vi "IntegerTester.vi"() -> ()   [LabVIEW 2017]
panel:
  out "RandomTestingthing":i32
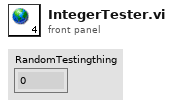
[diagram p1: front panel]
diagram:
